vi "Half Adder.vi"(8 "B":bool, 11 "A":bool) -> (0 "Carry":bool, 3 "Sum":bool)   [LabVIEW 2016]
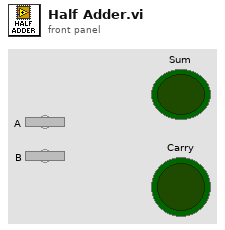
[diagram p1: front panel]
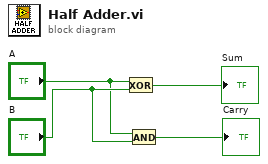
[diagram p0: block diagram]
diagram:
  n1 = Exclusive Or(1:"B", 2:"A") -> (0:→"Sum":bool)
  n2 = And(x="A", y="B") -> (x .and. y?=→"Carry":bool)
